vi "Read Sequence.vi"(8 "error in (no error)":errorcluster, 9 "Channel Mask":u64, 10 "Config Data":T3, 11 "Connection Data In":T2) -> (0 "error out":errorcluster, 1 "Adquisition Data Out":T1, 3 "Connection Data Out":T2)   [LabVIEW 2014, in "MSX-E3711_dll.lvlib"]
doc: "Recibe el Channel mask y el Config data. Abre el puerto e inicia la adquisición de valores en forma secuencial. Al mismo tiempo lee el estado de las I/O."
uses:
  MSX-E3711_dll.lvlib
  Typedef/Config Data.ctl
  Typedef/Connection Data.ctl
  E:/Repositorio Magnis/INF002/v0/Modules/HAL/Drivers/Sync/ADDI-DATA MSX-E3711/API/MSXE371x.dll
  MSXE371x.dll
  E:/Repositorio Magnis/INF002/v0/Modules/HAL/Drivers/Sync/ADDI-DATA MSX-E3711/API/MXCommon.dll
  MXCommon.dll
  Typedef/Adquisition Data.ctl
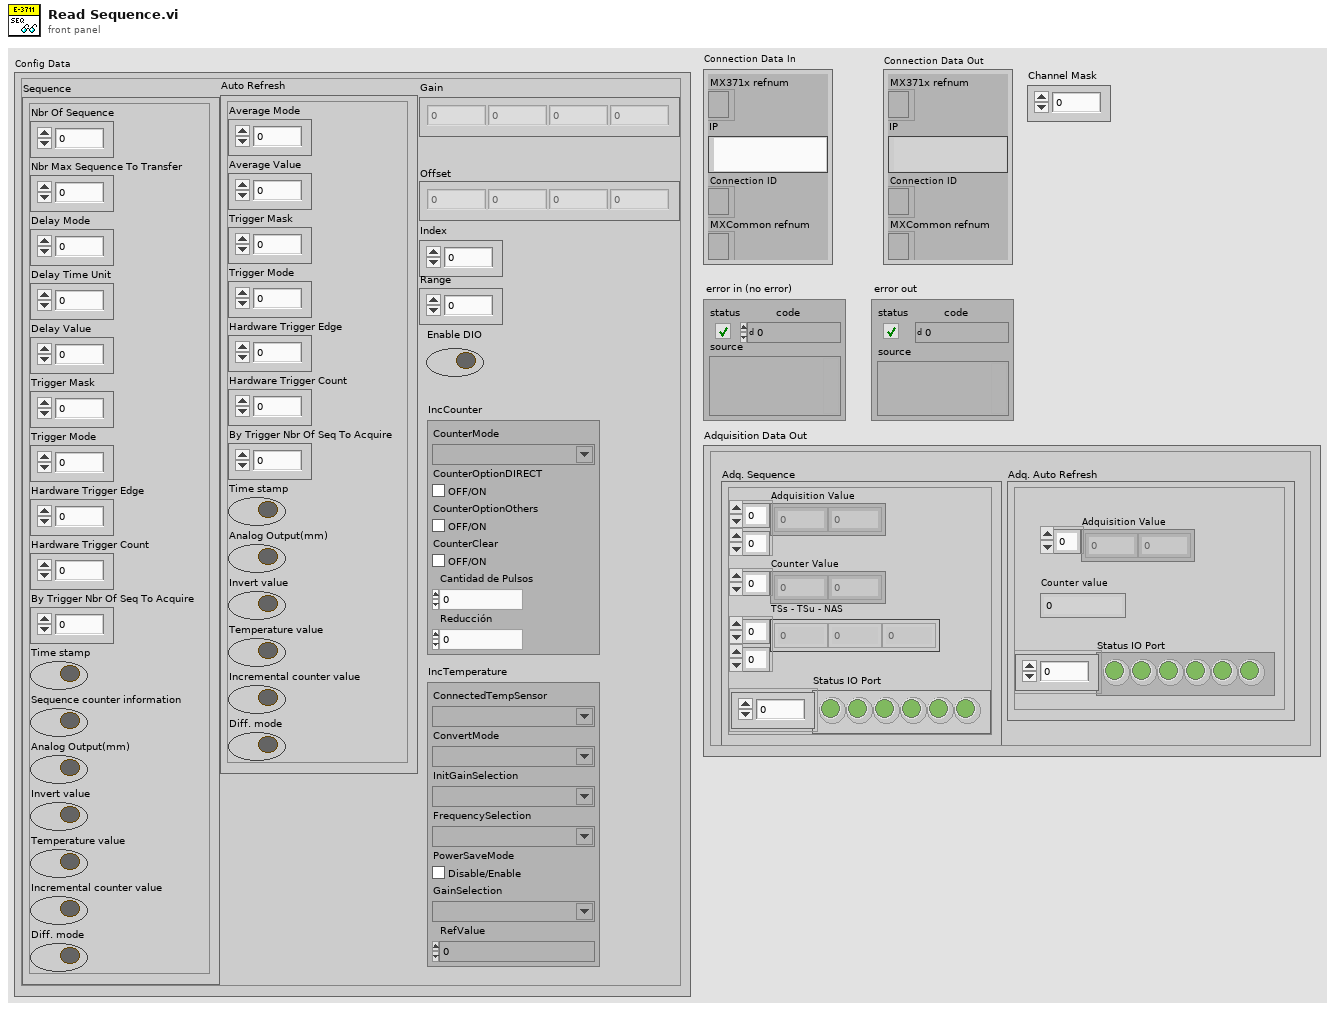
[diagram p1: front panel]
types:
  T1 = typedef "MSX-E3711_dll.lvlib/Adquisition Data.ctl" = cluster{"Adq. Sequence":cluster{"Adquisition Value":u32[][], "Counter Value":u32[], "TSs - TSu - NAS":u64[][], "Status IO Port":bool[]}, "Adq. Auto Refresh":cluster{"Adquisition Value":u64[], "Status IO Port":bool[], "Counter value":u32}}
  T2 = typedef "MSX-E3711_dll.lvlib/Connection Data.ctl" = cluster{"MX371x refnum":refnum<k24>, "IP":string, "Connection ID ":refnum<k5>, "MXCommon refnum":refnum<k24>}
  T3 = typedef "MSX-E3711_dll.lvlib/Config Data.ctl" = cluster{"Auto Refresh":cluster{"Average Mode":u64, "Average Value":u64, "Trigger Mask":u64, "Trigger Mode":u64, "Hardware Trigger Edge":u64, "Hardware Trigger Count":u64, "By Trigger Nbr Of Seq To Acquire":u64, "Time stamp":bool, "Analog Output(mm)":bool, "Invert value":bool, "Temperature value":bool, "Incremental counter value":bool, "Diff. mode":bool}, "Gain":sgl[], "Offset":sgl[], "Index":u64, "Range":sgl, "Sequence":cluster{"Nbr Of Sequence":u64, "Nbr Max Sequence To Transfer":u64, "Delay Mode":u64, "Delay Time Unit":u64, "Delay Value":u64, "Trigger Mask":u64, "Trigger Mode":u64, "Hardware Trigger Edge":u64, "Hardware Trigger Count":u64, "By Trigger Nbr Of Seq To Acquire":u64, "Time stamp":bool, "Sequence counter information":bool, "Analog Output(mm)":bool, "Invert value":bool, "Temperature value":bool, "Incremental counter value":bool, "Diff. mode":bool}, "Enable DIO":bool, "IncCounter":cluster{"CounterMode":string, "CounterOptionDIRECT  ":bool, "CounterOptionOthers":bool, "CounterClear ":bool, "Cantidad de Pulsos":sgl, "Reducción":sgl}, "IncTemperature":cluster{"ConnectedTempSensor":string, "ConvertMode":string, "InitGainSelection":string, "FrequencySelection":string, "PowerSaveMode":bool, "GainSelection":string, "RefValue":dbl}}
  T4 = cluster{"Nbr Of Sequence":u64, "Nbr Max Sequence To Transfer":u64, "Delay Mode":u64, "Delay Time Unit":u64, "Delay Value":u64, "Trigger Mask":u64, "Trigger Mode":u64, "Hardware Trigger Edge":u64, "Hardware Trigger Count":u64, "By Trigger Nbr Of Seq To Acquire":u64, "Time stamp":bool, "Sequence counter information":bool, "Analog Output(mm)":bool, "Invert value":bool, "Temperature value":bool, "Incremental counter value":bool, "Diff. mode":bool}
  T5 = enum16{"big-endian, network order", "native, host order", "little-endian"}
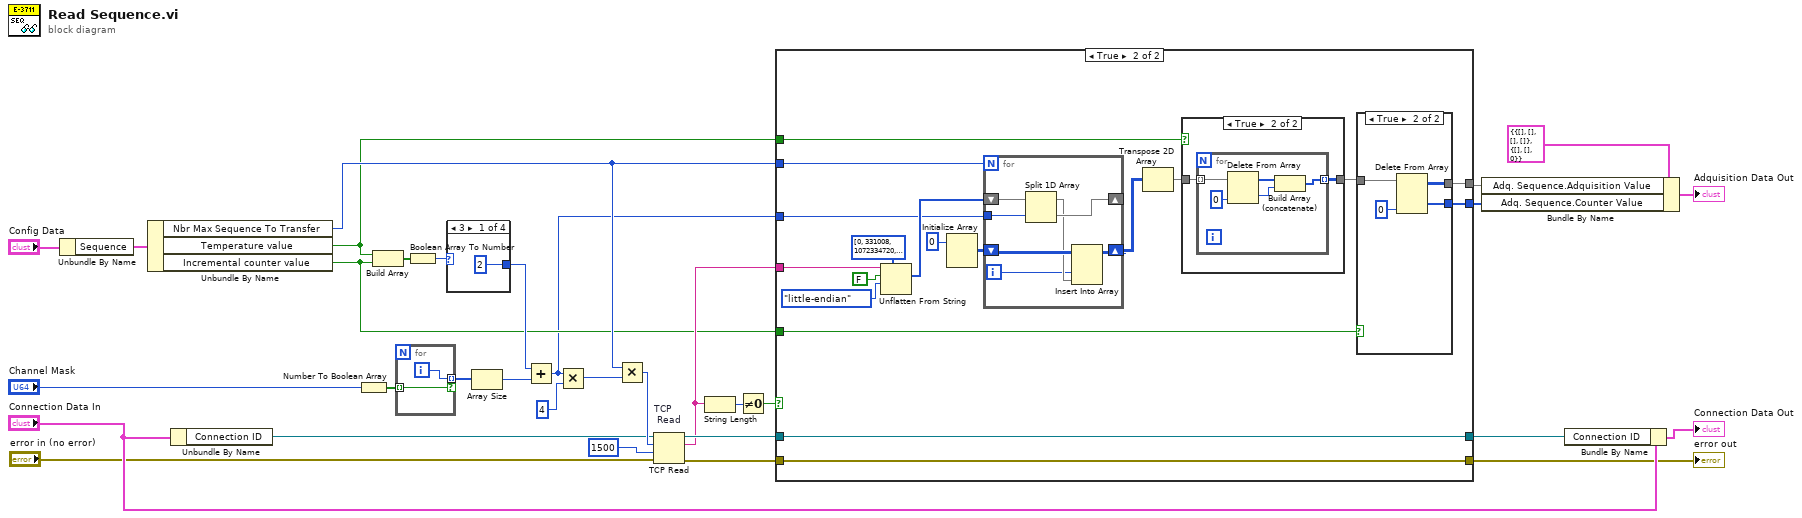
[diagram p0: block diagram]
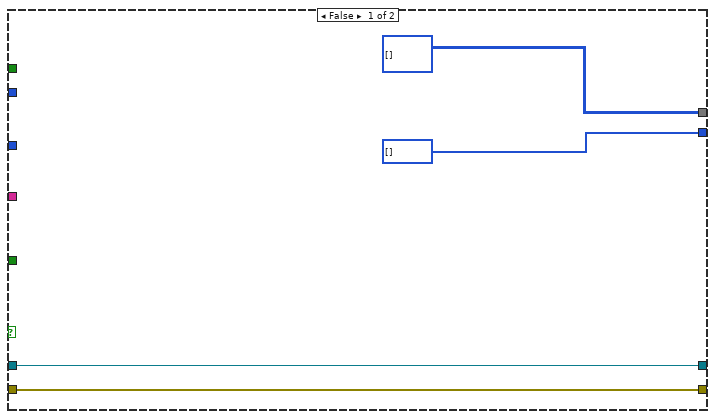
[diagram p2: hidden frame]
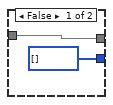
[diagram p3: hidden frame]
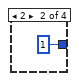
[diagram p5: hidden frame]
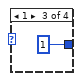
[diagram p6: hidden frame]
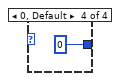
[diagram p7: hidden frame]
diagram:
  n1 = Unbundle By Name("Config Data") -> ("Sequence"=w29:T4)
  n2 = Unbundle By Name(w29) -> ("Nbr Max Sequence To Transfer"=w11:u64, "Temperature value"=w5:bool, "Incremental counter value"=w6:bool)
  n3 = Unbundle By Name("Connection Data In") -> ("Connection ID"=w17:refnum<k5>)
  n4 = Number To Boolean Array(number="Channel Mask") -> (Boolean array=w31:bool[])
  n5 = Build Array(w5, w6) -> (w21:bool[])
  n6 = for {
    tunnel: [w34] -> w30 mode=indexing if=w33
    tunnel: w31 -> [w33] mode=indexing
    i -> [w34]
  }
  n7 = Boolean Array To Number(Boolean array=w21) -> (number=w20:u32)
  n8 = case shown="3" w20 {
    tunnel: [2 1 1 0] -> w16
    frame 3 {
    }
    frame 2 {
    }
    frame 1 {
    }
    frame 0, Default {
    }
  }
  n9 = Array Size(array=w30) -> (size(s)=w7:i32)
  n10 = Add(x=w16, y=w7) -> (x+y=w1:i32)
  n11 = Multiply(x=w1, y=4) -> (x*y=w10:i32)
  n12 = Multiply(x=w11, y=w10) -> (x*y=w28:u64)
  n13 = TCP Read "TCP\n Read"(connection ID=w17, bytes to read=w28, error in (no error)="error in (no error)", 9:1500 ("timeout ms (25000)")) -> (connection ID out=w15:refnum<k5>, data out=w12:string, error out=w14:errorcluster)  [unwired: 1 in]
  n14 = String Length(string=w12) -> (length=w24:i32)
  n15 = Not Equal To 0?(x=w24) -> (x != 0?=w13:bool)
  n16 = case shown="True" w13 {
    tunnel: w12 -> [_ w58]
    tunnel: w14 -> [w42 w57]
    tunnel: [w42 w57] -> w8
    tunnel: w11 -> [_ w44]
    tunnel: w1 -> [_ w45]
    tunnel: [w41 w56] -> w9
    tunnel: w15 -> [w41 w56]
    tunnel: w5 -> [_ w54]
    tunnel: w6 -> [_ w53]
    tunnel: [u32[][] [] w51] -> w4
    tunnel: [u32[] [] w50] -> w3
    frame False {
    }
    frame True {
      n17 = Unflatten From String(type=u32[] [0, 331008, 1072334720, 3195303168, 4729, 331808, 1072334336, 3195309312, 4729, 332608, 1072334080, 3195300096, 4729, 333408, 1072334400, 3195303936, 4729, 334208, 1072334336, 3195305728, 4729, 335008, 1072334400, 3195309568, 4729, 335808, 1072334912, 3195305472, 4729, 336608, 1072333568, 3195304704, 4729, 337408, 1072333440, 3195311872, 4729, 338208, 1072334720, 3195307264, 4729, 339008, 1072334272, 3195311616, 4729, 339808, 1072334272, 3195305984, 4729, 340608, 1072334400, 3195307776, 4729, 341408, 1072334080, 3195308288, 4729, 342208, 1072334720, 3195304448, 4729, 343008, 1072335488, 3195307264, 4729, 343808, 1072334080, 3195302912, 4729, 344608, 1072334272, 3195311360, 4729, 345408, 1072334848, 3195309056, 4729, 346208, 1072334784, 3195301376, 4729, 347008, 1072335168, 3195305472, 4729, 347808, 1072334912, 3195314688, 4729, 348608, 1072334080, 3195299584, 4729, 349408, 1072334144, 3195304448, 4729, 350208, 1072334400, 3195304448, 4729, 351008, 1072335296, 3195304960, 4729, 351808, 1072334144, 3195309824, 4729, 352608, 1072334784, 3195303168, 4729, 353408, 1072334464, 3195305472, 4729, 354208, 1072335168, 3195313920, 4729, 355008, 1072334400, 3195304960, 4729, 355808, 1072334144, 3195304192, 4729, 356608, 1072334528, 3195307776, 4729, 357408, 1072335104, 3195309056, 4729, 358208, 1072333824, 3195308544, 4729, 359008, 1072334208, 3195309312, 4729, 359808, 1072334272, 3195306240, 4729, 360608, 1072334848, 3195309312, 4729, 361408, 1072334656, 3195302912, 4729, 362208, 1072334528, 3195305216, 4729, 363008, 1072334528, 3195304192, 4729, 363808, 1072335232, 3195316480, 4729, 364608, 1072334784, 3195305216, 4729, 365408, 1072333824, 3195308800, 4729, 366208, 1072334784, 3195309312, 4729, 367008, 1072334784, 3195302656, 4729, 367808, 1072333632, 3195310336, 4729, 368608, 1072333568, 3195305984, 4729, 369408, 1072334336, 3195305728, 4729, 370208, 1072334656, 3195304448, 4729, 371008, 1072334208, 3195305984, 4729, 371808, 1072334336, 3195306240, 4729, 372608, 1072334144, 3195302656, 4729, 373408, 1072334592, 3195300864, 4729, 374208, 1072334016, 3195302400, 4729, 375008, 1072334144, 3195307264, 4729, 375808, 1072334528, 3195312640, 4729, 376608, 1072334784, 3195302400, 4729, 377408, 1072333696, 3195305728, 4729, 378208, 1072334656, 3195302144, 4729, 379008, 1072334464, 3195306752, 4729, 379808, 1072334272, 3195306496, 4729, 380608, 1072334272, 3195307776, 4729, 381408, 1072334400, 3195306496, 4729, 382208, 1072334592, 3195300608, 4729, 383008, 1072334400, 3195303168, 4729, 383808, 1072334016, 3195304192, 4729, 384608, 1072334016, 3195309568, 4729, 385408, 1072334912, 3195306496, 4729, 386208, 1072334656, 3195303424, 4729, 387008, 1072334080, 3195302912, 4729, 387808, 1072334592, 3195309312, 4729, 388608, 1072334272, 3195299072, 4729, 389408, 1072334144, 3195304704, 4729, 390208, 1072334272, 3195304960, 4729, 391008, 1072334144, 3195305472, 4729, 391808, 1072334336, 3195301632, 4729, 392608, 1072334464, 3195307008, 4729, 393408, 1072334016, 3195311616, 4729, 394208, 1072335168, 3195310336, 4729, 395008, 1072335232, 3195308288, 4729, 395808, 1072334592, 3195303680, 4729, 396608, 1072334016, 3195308288, 4729, 397408, 1072335296, 3195304448, 4729, 398208, 1072334400, 3195310080, 4729, 399008, 1072334464, 3195302912, 4729, 399808, 1072334848, 3195305728, 4729, 400608, 1072334464, 3195306752, 4729, 401408, 1072334272, 3195306240, 4729, 402208, 1072334656, 3195305216, 4729, 403008, 1072334272, 3195307008, 4729, 403808, 1072335296, 3195315968, 4729, 404608, 1072334336, 3195302656, 4729, 405408, 1072334336, 3195304192, 4729, 406208, 1072334528, 3195309568, 4729, 407008, 1072334912, 3195303168, 4729, 407808, 1072333952, 3195309312, 4729, 408608, 1072334272, 3195307520, 4729, 409408, 1072334464, 3195306496, 4729, 410208, 1072334400, 3195305472] ("Array - Numeric"), binary string=w58, data includes array or string size? (T)=FALSE, byte order (0:big-endian, network order)=T5."little-endian") -> (value=w46:u32[])  [unwired: 1 in, 2 out]
      n18 = Initialize Array(u32 0 ("element")) -> (w47:u32[][])  [unwired: 2 in]
      n19 = for {
        N: w44 -> [_]
        shift-right: [w65] -> _
        shift-left: w46 -> [w67]
        tunnel: w45 -> [w66]
        shift-right: [w63] -> w49
        shift-left: w47 -> [w64]
        i -> [w61]
        n20 = Split 1D Array(array=w67, index=w66) -> (first subarray=w62:u32[], second subarray=w65:u32[])
        n21 = Insert Into Array(array=w64, index (col)=w61, new element=w62) -> (w63:u32[][])  [unwired: 1 in]
      }
      n22 = Transpose 2D Array(2D array=w49) -> (transposed array=w43:u32[][])
      n23 = case shown="True" w54 {
        tunnel: [w74 w75] -> w52
        tunnel: w43 -> [w74 w76]
        frame False {
        }
        frame True {
          n24 = for {
            tunnel: w76 -> [w81] mode=indexing
            tunnel: [w80] -> w75 mode=indexing
            n25 = Delete From Array(array=w81, index=0 ("disabled index (col)")) -> (deleted portion=w79:u32, array with subset deleted=w78:u32[])  [unwired: 1 in]
            n26 = Build Array (concatenate)(w78, w79) -> (w80:u32[])
          }
        }
      }
      n27 = case shown="True" w53 {
        tunnel: [w69 w70] -> w51
        tunnel: w52 -> [w69 w72]
        tunnel: [u32[] [] w71] -> w50
        frame False {
        }
        frame True {
          n28 = Delete From Array(array=w72, index (col)=0 ("disabled index (col)")) -> (deleted portion=w71:u32[], array with subset deleted=w70:u32[][])  [unwired: 2 in]
        }
      }
    }
  }
  "error out" <- w8
  n29 = Bundle By Name(cluster=T1 {"Adq. Sequence"={"Adquisition Value"=[], "Counter Value"=[], "TSs - TSu - NAS"=[], "Status IO Port"=[]}, "Adq. Auto Refresh"={"Adquisition Value"=[], "Status IO Port"=[], "Counter value"=0}} ("Adquisition Data Out 2"), "Adq. Sequence.Adquisition Value"=w4, "Adq. Sequence.Counter Value"=w3) -> (→"Adquisition Data Out":T1)
  n30 = Bundle By Name(cluster="Connection Data In", "Connection ID"=w9) -> (→"Connection Data Out":T2)
